vi "SignalGenerator(SubVI).vi"(8 "error in (no error)":errorcluster, 9 "Stop":bool, 10 "Amplitude":dbl, 11 "Frequency":dbl) -> (0 "error out":errorcluster)   [LabVIEW 2015]
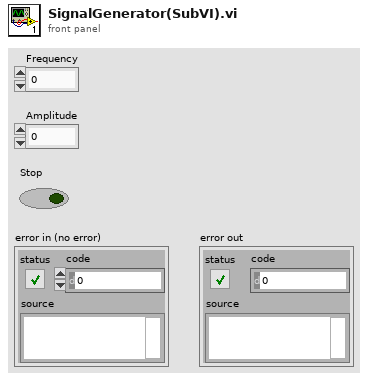
[diagram p1: front panel]
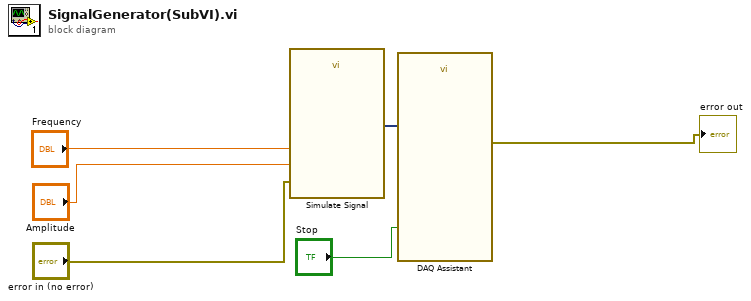
[diagram p0: block diagram]
diagram:
  n1 = call "Simulate Signal"("Frequency"="Frequency", "Amplitude"="Amplitude", "error in (no error)"="error in (no error)") -> ("Sine"=w2:dynamicdata)  [unwired: 11 in, 1 out]
  n2 = call "DAQ Assistant"("data"=w2, "stop (F)"="Stop") -> ("error out"=→"error out":errorcluster)  [unwired: 15 in, 2 out]
